vi "ni_to_range.vi"(1 "end":dbl, 2 "start":dbl, 3 "i":i32, 4 "N":i32) -> (0 "current value (runs from start to end in N steps)":dbl)   [LabVIEW 2010]
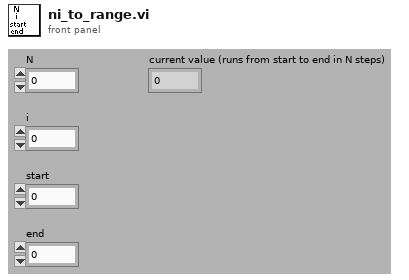
[diagram p1: front panel]
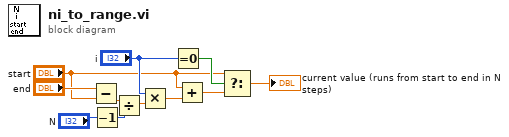
[diagram p0: block diagram]
diagram:
  n1 = Subtract(x="end", y="start") -> (x-y=w8:dbl)
  n2 = Decrement(x="N") -> (x-1=w9:i32)
  n3 = Divide(x=w8, y=w9) -> (x/y=w10:dbl)
  n4 = Multiply(x="i", y=w10) -> (x*y=w11:dbl)
  n5 = Equal To 0?(x="i") -> (x = 0?=w2:bool)
  n6 = Add(x="start", y=w11) -> (x+y=w3:dbl)
  n7 = Select(t="start", s=w2, f=w3) -> (s? t:f=→"current value (runs from start to end in N steps)":dbl)
